vi "Test_ListAll_EmptyTable_ReturnEmpty.vi"(8 "error in (no error)":errorcluster, 11 "TestCase in":refnum<class "TestComposedLookupTable.lvclass">) -> (0 "error out":errorcluster, 3 "TestCase out":refnum<class "TestComposedLookupTable.lvclass">)   [LabVIEW 2017, in "TestComposedLookupTable.lvclass"]
uses:
  TestComposedLookupTable.lvclass
  Source/LookupTable/LookupTable.lvclass/LookupTable.ctl
  Source/LookupTable/Read Table Reference.vi
  Source/LookupTable/LookupTable.lvclass
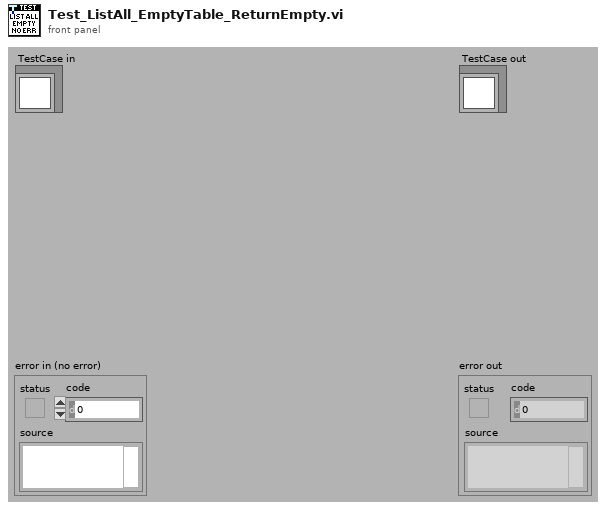
[diagram p1: front panel]
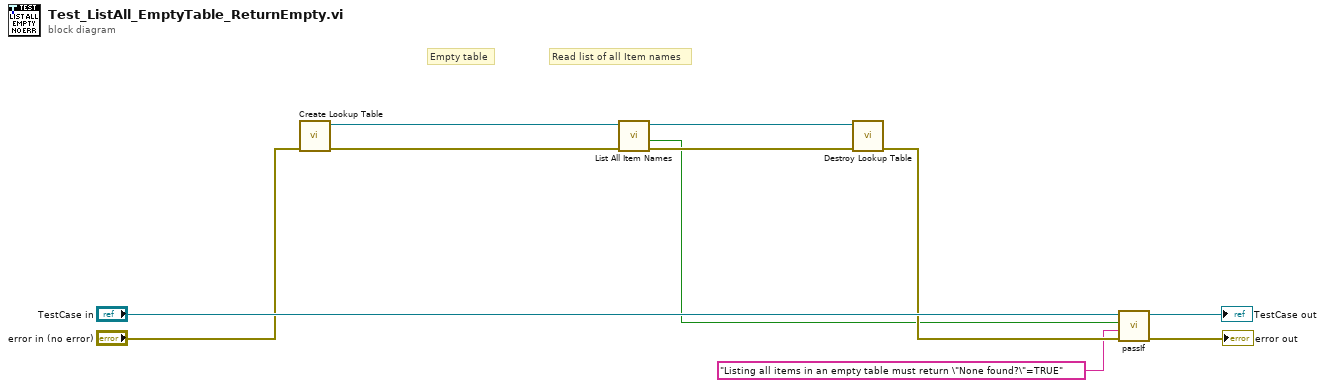
[diagram p0: block diagram]
diagram:
  # "Empty table"
  # "Read list of all Item names"
  n1 = call "Create Lookup Table.vi"("error in (no error)"="error in (no error)") -> ("error out"=w11:errorcluster, "LookupTable Reference"=w7:refnum<data-value>)  [unwired: 9 in]
  n2 = call "List All Item Names.vi"("error in (no error)"=w11, "LookupTable Reference"=w7) -> ("error out"=w4:errorcluster, "None Found?"=w2:bool, "LookupTable Reference Out"=w3:refnum<data-value>)  [unwired: 6 in, 1 out]
  n3 = call "Destroy Lookup Table.vi"("error in (no error)"=w4, "LookupTable Reference"=w3) -> ("error out"=w5:errorcluster)  [unwired: 9 in]
  n4 = call-dynamic "passIf.vi"("error in (no error)"=w5, "message (\"\")"="Listing all items in an empty table must return \"None found?\"=TRUE" ("message (\"\")"), "pass"=w2, "TestCase in"="TestCase in") -> ("error out"=→"error out":errorcluster, "TestCase out"=→"TestCase out":refnum<class "TestComposedLookupTable.lvclass">)  [unwired: 6 in]
